vi "WriteToFIFO.vi"() -> ()   [LabVIEW 2011]
uses:
  <vilib>/rvi/eio/common/nirviEmuTemplateMethod_errors.vi
  <vilib>/rvi/interface/RandomDataEmulation/nirviRandomDataFPGAFIFO.vi
  <vilib>/rvi/interface/RandomDataEmulation/niFpgaRandomDataHandleErrors.vi
  <vilib>/eio/EIONode/EIONode.xnode
  <vilib>/eio/EIOMethodNode/EIOMethodNode.xnode
  <vilib>/rvi/DataTransferAndStorage/Container/XNode/niFpgaContainer.xnode
  <vilib>/rvi/interface/RandomDataEmulation/nirviRandomDataFpgaReadWriteTemplate.vi
panel:
  in  "stop":bool
  out "Numeric":i32
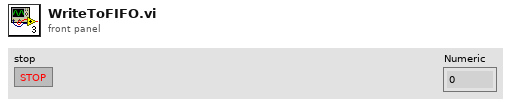
[diagram p1: front panel]
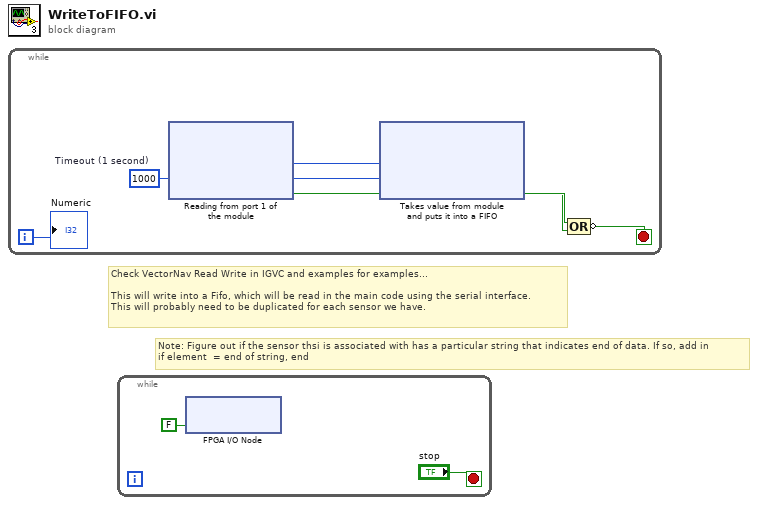
[diagram p0: block diagram]
diagram:
  # "Note: Figure out if the sensor thsi is associated with has a particular string that indicates end of data. If so, add in\nif element  = end of string, end"
  # "Check VectorNav Read Write in IGVC and examples for examples...\n\nThis will write into a Fifo, which will be read in the main code using the serial interface.\nThis will probably need to be duplicated for each sensor we have."
  n1 = while {
    i -> [w1]
    stop <- w2 stop-if-true
    w3 = 1000  # Timeout (1 second)
    n2 = xnode "Reading from port 1 of the module"("Timeout (ms)"=w3) -> ("Data"=w6:u8, "Timed Out"=w4:bool)  [unwired: 1 in, 1 out]
    n3 = xnode "Takes value from module and puts it into a FIFO"("Element"=w6, "Timeout"=w3) -> ("Timed Out?"=w5:bool)  [unwired: 1 in, 1 out]
    n4 = Compound Arithmetic op=OR(w5, w4) -> (invert w2:bool)
    "Numeric" <- w1
  }
  n5 = while {
    stop <- "stop" stop-if-true
    n6 = xnode "FPGA I/O Node"("FPGA LED"=FALSE) -> ()  [unwired: 1 in, 1 out]
  }
